vi "RIB Req - UDP Enable UPS.vi"(0 "Limits File Path":path, 5 "Results File Path":path, 11 "error in":errorcluster) -> (4 "Results Data Array":string[][](array[string]), 15 "error out":errorcluster)   [LabVIEW 2024]
doc: "Template test"
uses:
  <vilib>/addons/_JKI Toolkits/State Machine/_JKI_lib_State_Machine.llb/Select State(s)_err__jki_lib_state_machine.vi
  <vilib>/addons/_JKI Toolkits/State Machine/_JKI_lib_State_Machine.llb/Select State(s)_bool__jki_lib_state_machine.vi
  <vilib>/addons/_JKI Toolkits/State Machine/_JKI_lib_State_Machine.llb/Periodic Trigger__ogtk__JKI-SM__jki_lib_state_machine.vi
  <userlib>/_OpenG.lib/file/file.llb/Strip Path Extension - String__ogtk.vi
  <vilib>/Utility/file.llb/Read Delimited Spreadsheet (string).vi
  <userlib>/_OpenG.lib/file/file.llb/openg_file.lvlib
  <userlib>/_OpenG.lib/appcontrol/appcontrol.llb/openg_application_control.lvlib
  <userlib>/_OpenG.lib/time/time.llb/openg_time.lvlib
  <vilib>/Utility/file.llb/Write Delimited Spreadsheet (string).vi
panel:
  in  "Connect":string
  in  "Connect Fail":string
  in  "Read Normal Operation":string
  in  "Read Wait for Start":string
  in  "Read TMS":string
  in  "Read ROV B":string
  in  "Read ROV A":string
  in  "5A Test":bool
  in  "task out":refnum<k21>
  out "Timeout (Read UDP)":dbl(slide) scale=0.0..20.0
  out "Results Data 2":string[](array[string])
  in  "UDP Read":string
  in  "connection ID":refnum<k16>
  in  "Exit":bool
  # "Enable UPS Test"
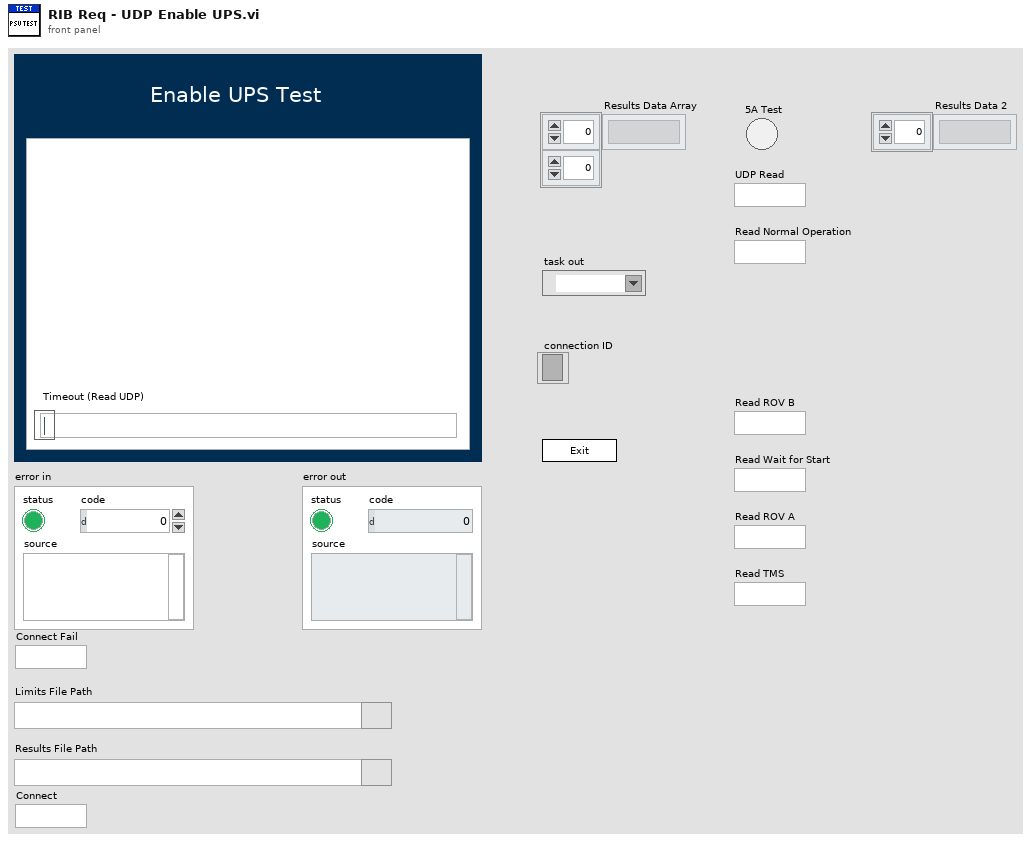
[diagram p1: front panel]
types:
  T1 = enum32{"Invalid", "Standard", "Closed", "Hidden", "Minimized", "Maximized"}
  T2 = enum32{"invalid app kind", "Development System", "Run Time System", "Student Edition", "Embedded LabVIEW", "Evaluation", "Custom"}
  T3 = typedef "FGV - Enum" = enum16{"Cleanup", "Get Data", "Open UDP", "Initialise DAQ", "Initialise I2C"}
  T4 = enum16{"Start Timer", "Get Time", "Pause", "Unpause"}
  T5 = cluster{"Core":cluster{"Current VI Reference":refnum<vi>, "Close Panel on Exit?":bool}, "Limits File Path":path, "Test Limits":string[][], "Results Data Array":string[][], "Results File Path":path, "UDP Read":string, "connection ID":refnum<k16>, "task out":refnum<k21>, "5A Test":bool, "Connect Fail":string, "Connect":string, "Read ROV A":string, "Read ROV B":string, "Read TMS":string, "Read Wait for Start":string, "Read Normal Operation":string}
  T6 = cluster{"Current VI Reference":refnum<vi>, "Close Panel on Exit?":bool}
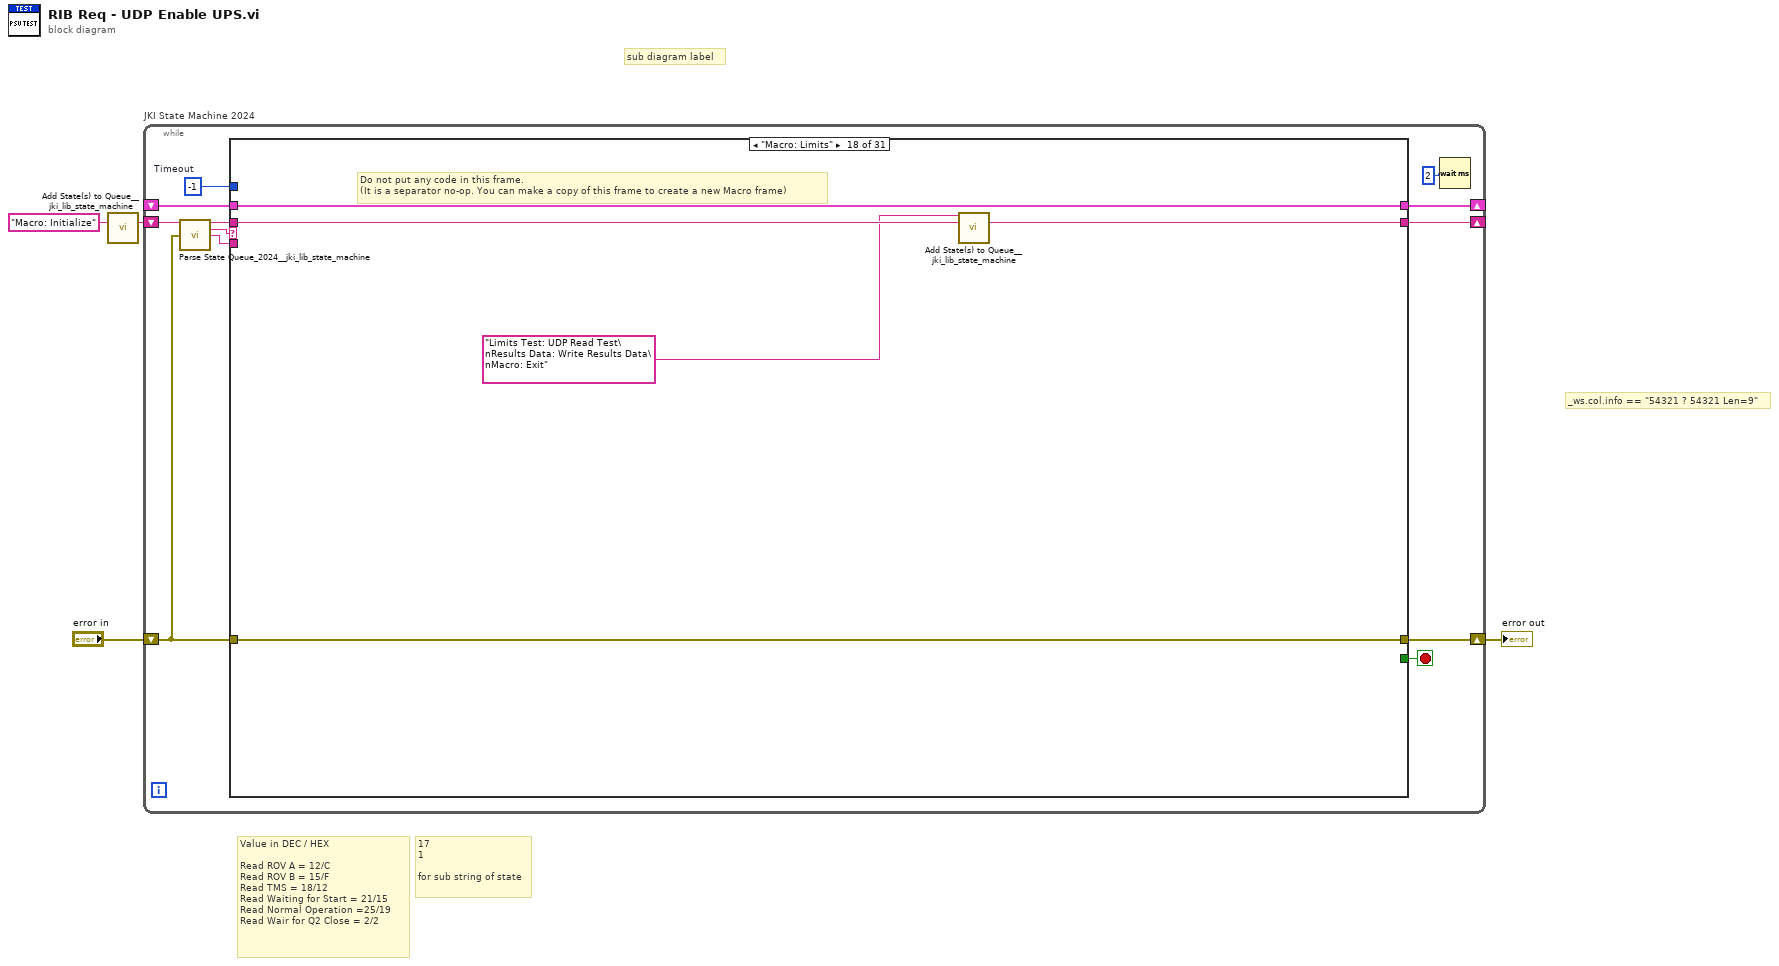
[diagram p0: block diagram]
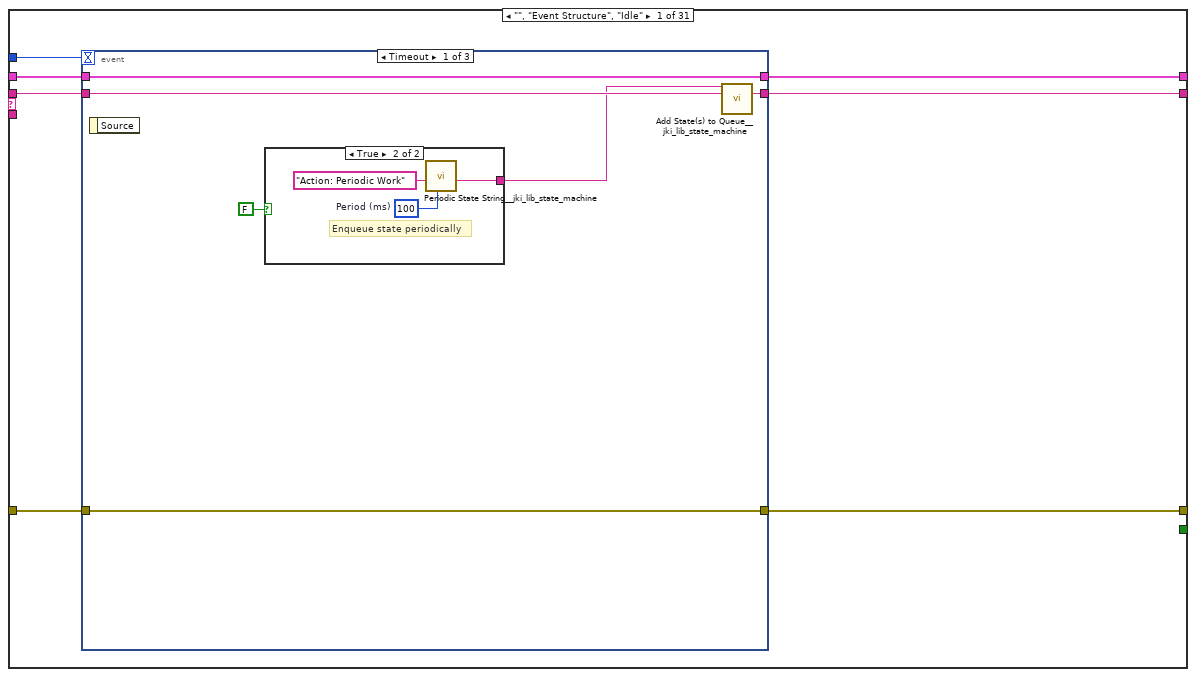
[diagram p2: hidden frame]
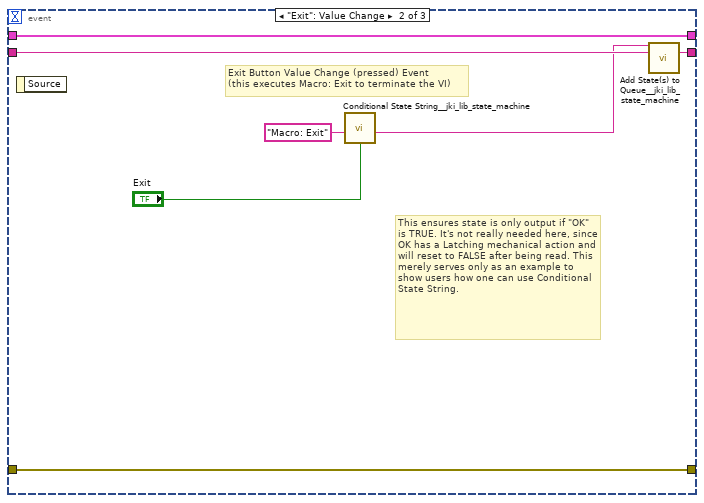
[diagram p4: hidden frame]
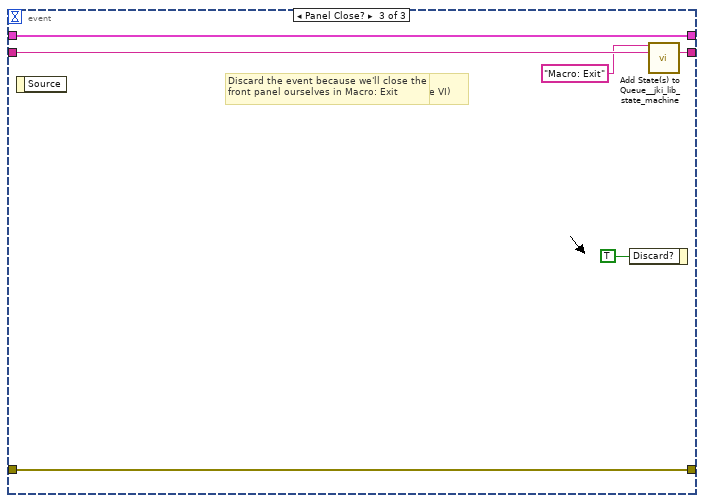
[diagram p5: hidden frame]
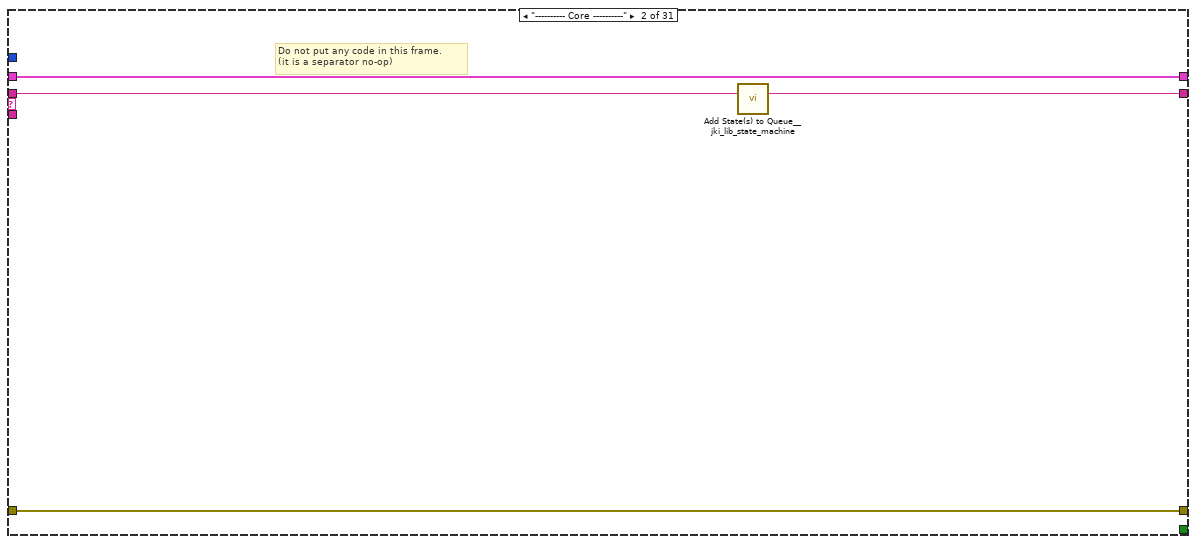
[diagram p6: hidden frame]
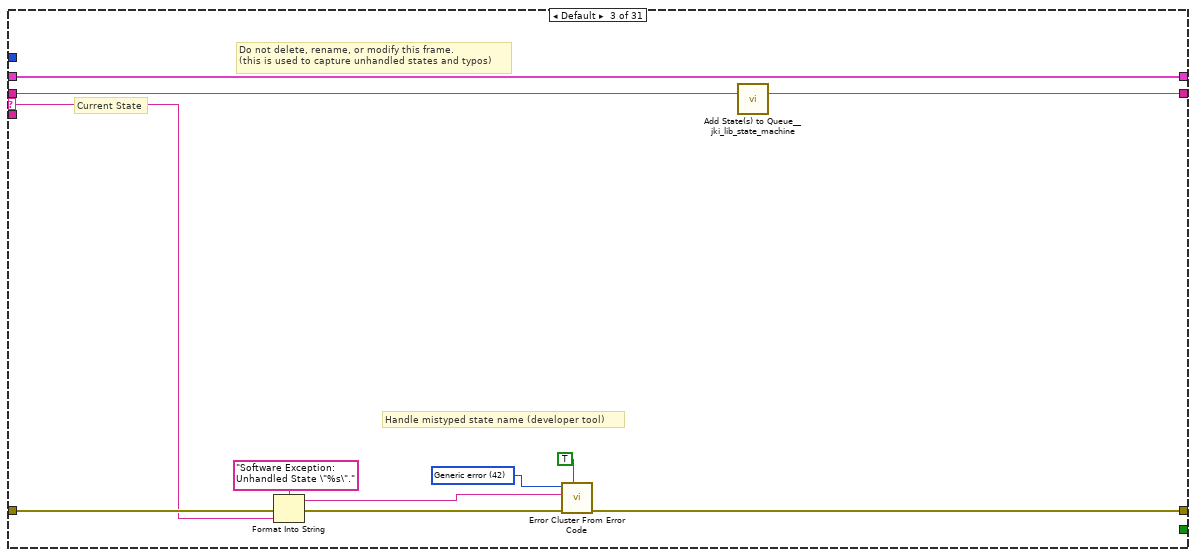
[diagram p7: hidden frame]
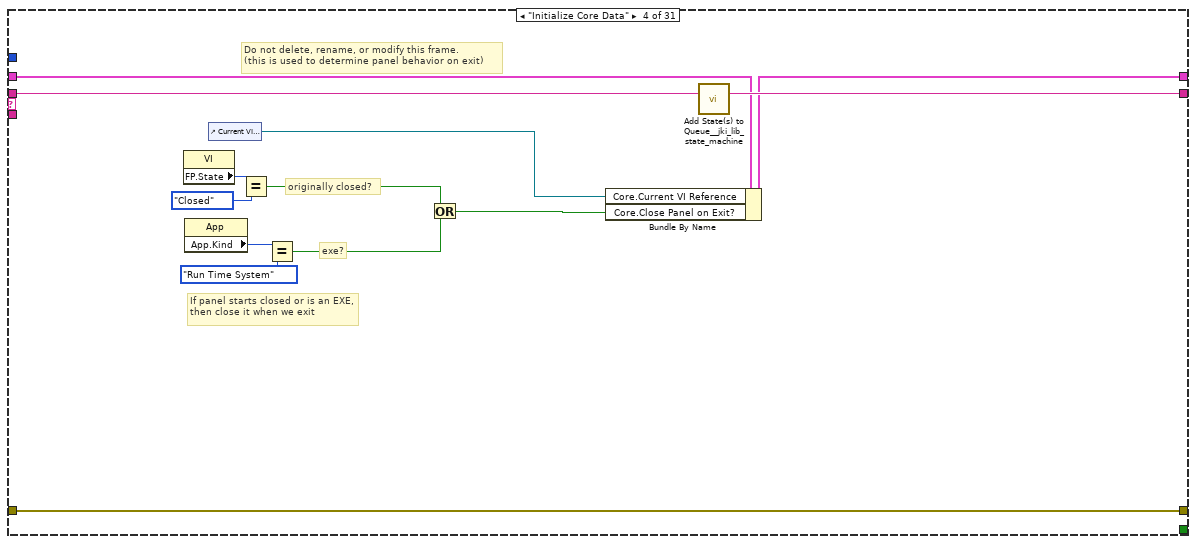
[diagram p8: hidden frame]
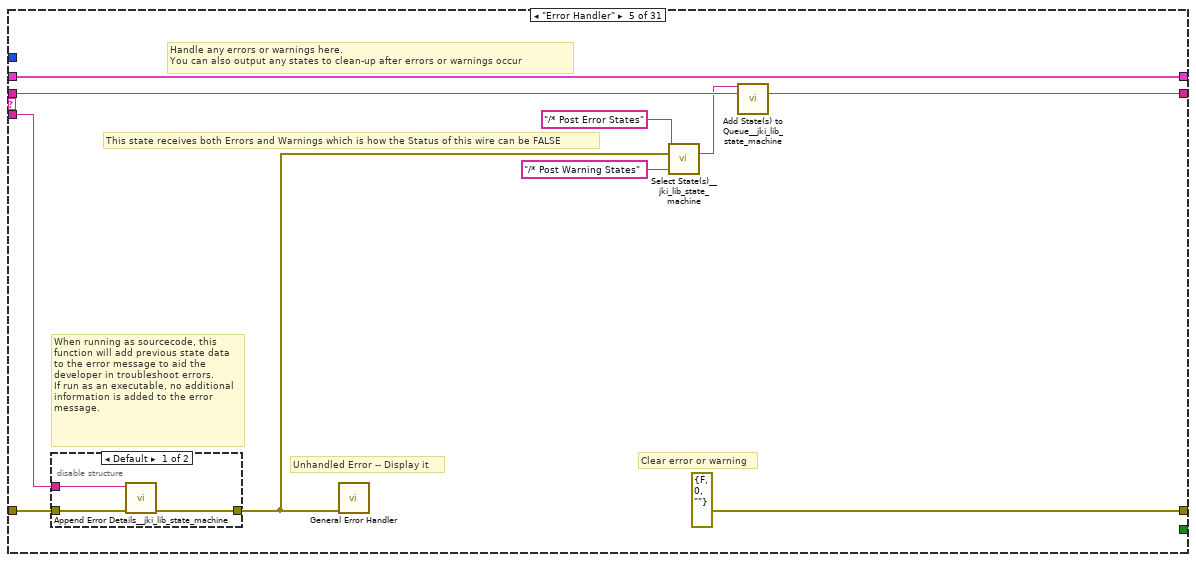
[diagram p9: hidden frame]
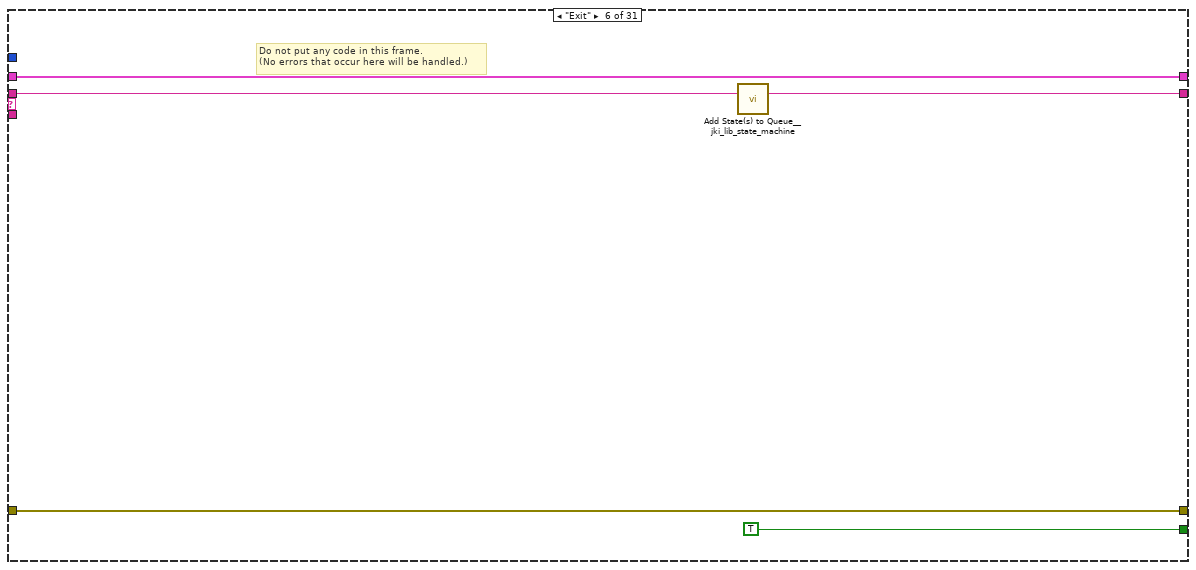
[diagram p11: hidden frame]
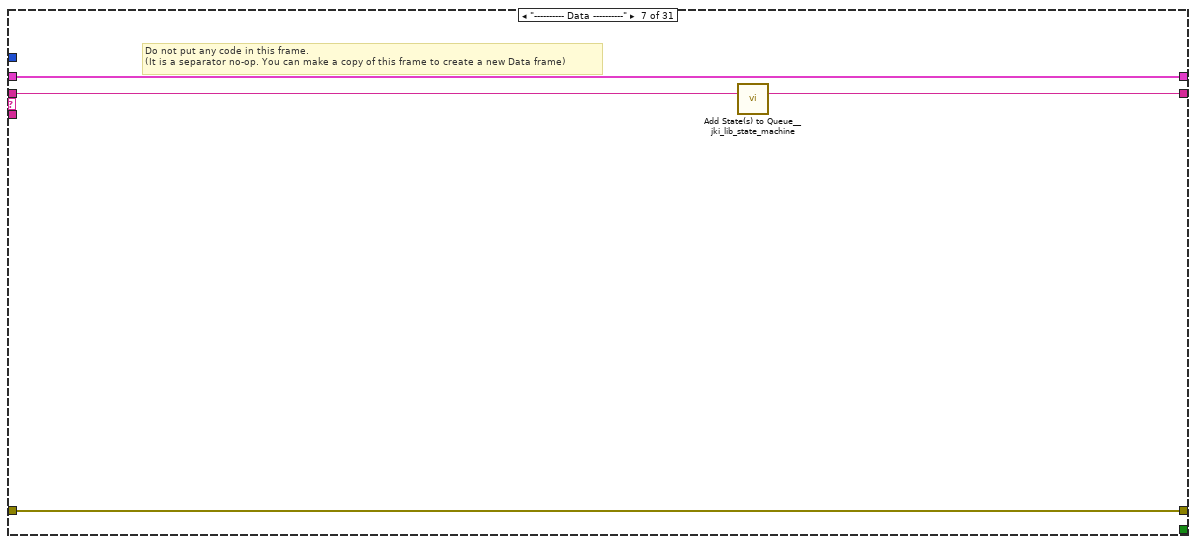
[diagram p12: hidden frame]
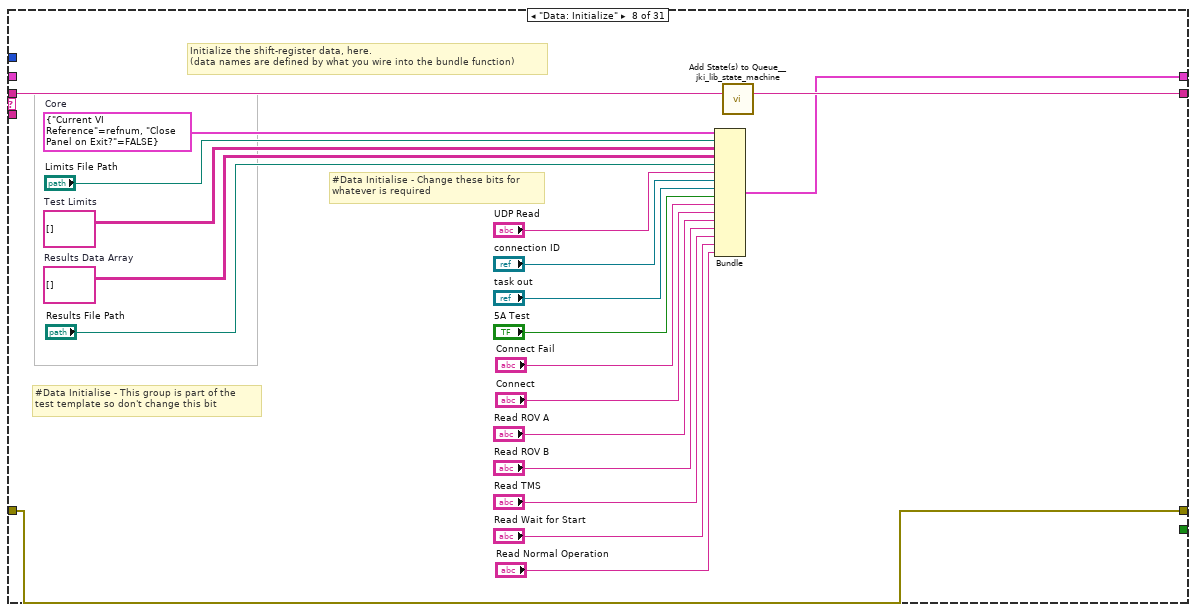
[diagram p13: hidden frame]
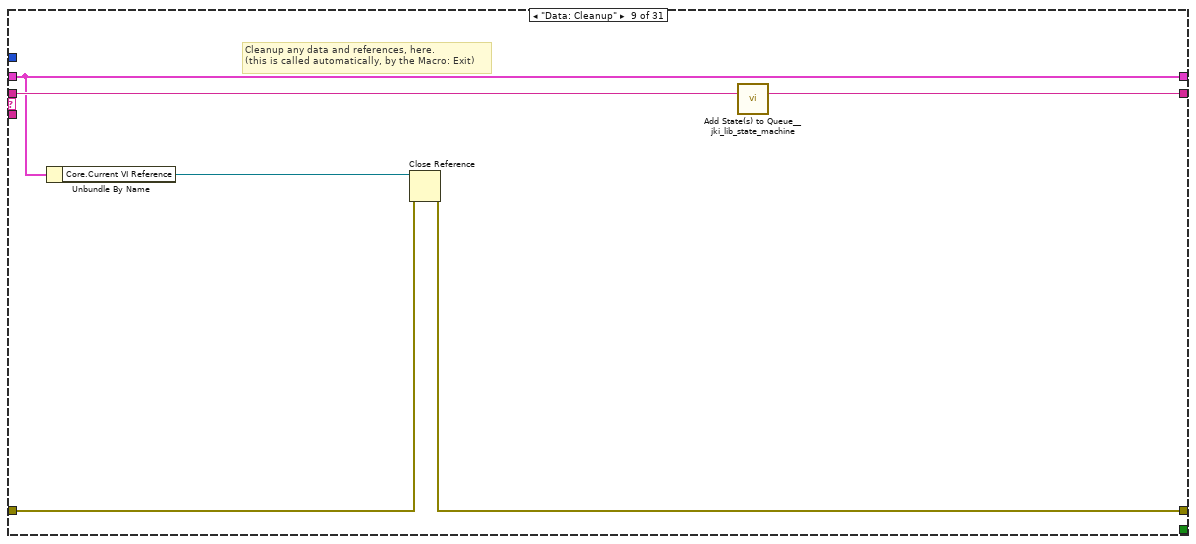
[diagram p14: hidden frame]
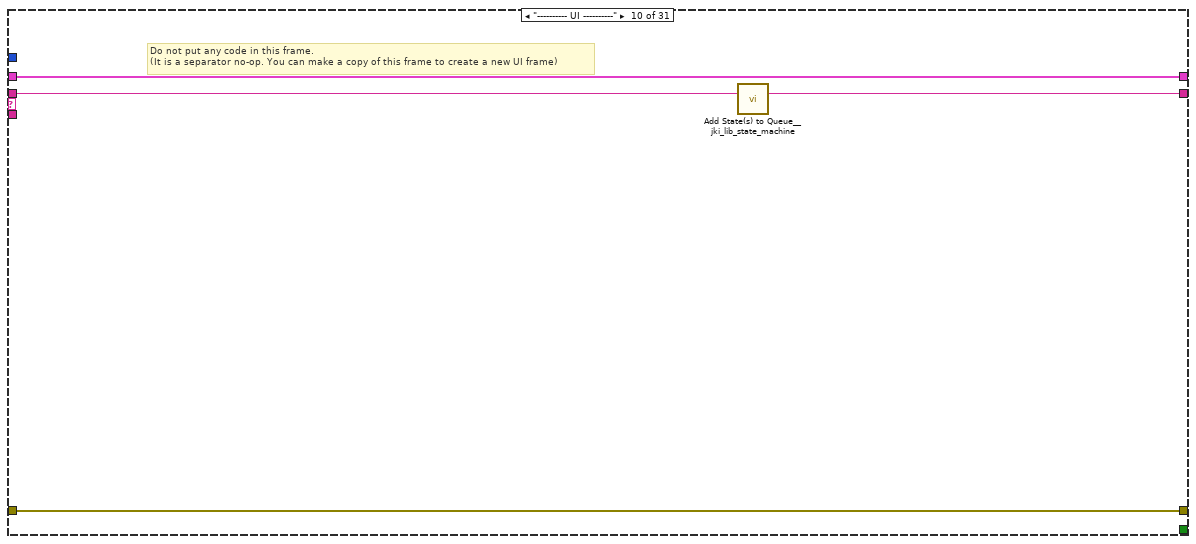
[diagram p15: hidden frame]
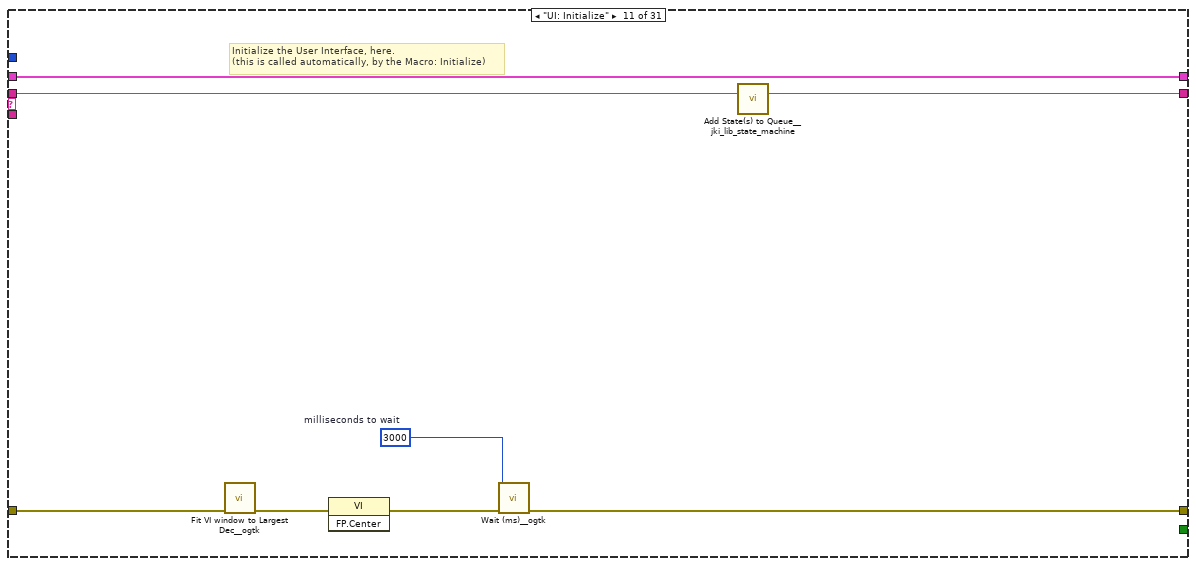
[diagram p16: hidden frame]
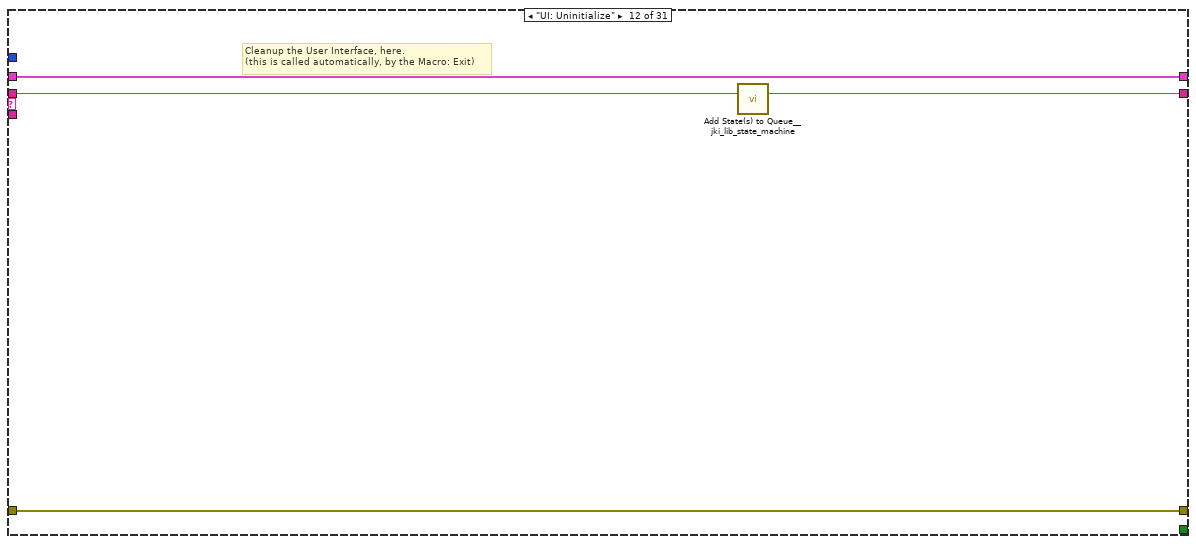
[diagram p17: hidden frame]
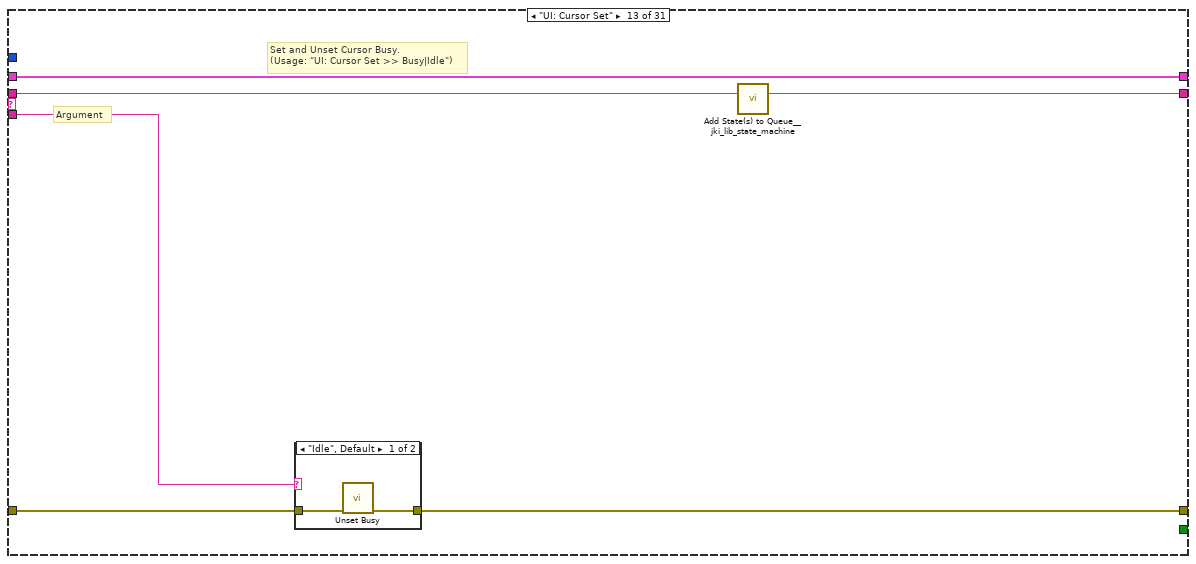
[diagram p18: hidden frame]
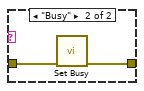
[diagram p19: hidden frame]
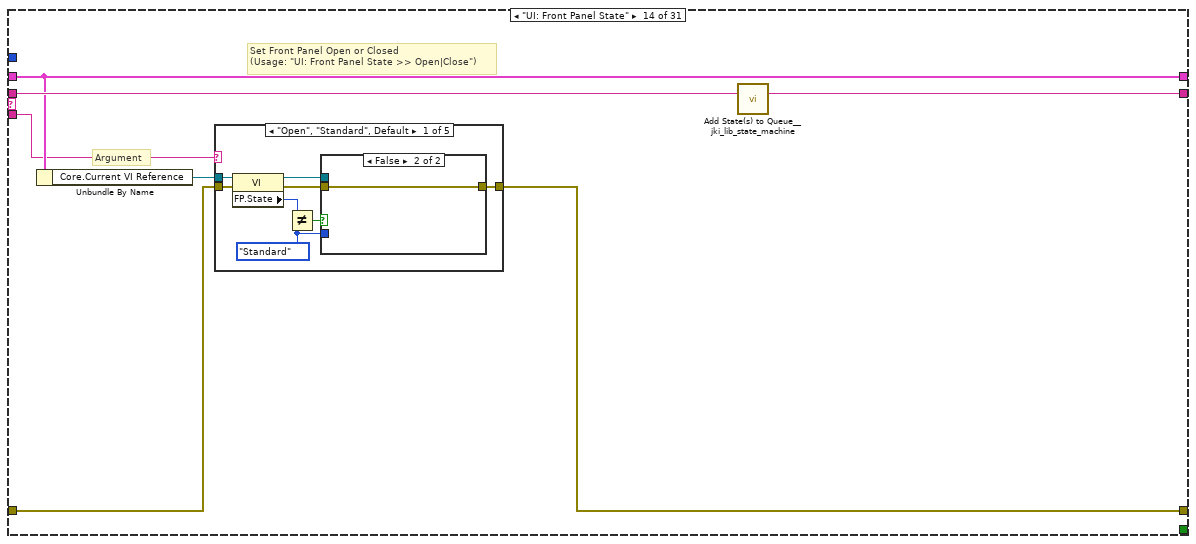
[diagram p20: hidden frame]
diagram:
  # "17\n1\n\nfor sub string of state"
  # "Value in DEC / HEX\n\nRead ROV A = 12/C\nRead ROV B = 15/F\nRead TMS = 18/12\nRead Waiting for Start = 21/15\nRead Normal Operation =25/19 \nRead Wair for Q2 Close = 2/2"
  # "_ws.col.info == \"54321 ? 54321 Len=9\""
  # "sub diagram label"
  n1 = call <vilib>:"Add State(s) to Queue__jki_lib_state_machine.vi"("State(s) in (\"\")"="Macro: Initialize") -> ("States Out"=w4:string)  [unwired: 14 in]
  n2 = while "JKI State Machine 2024" {
    shift-right: [w9] -> _
    shift-left: _ -> [w8]
    shift-right: [w12] -> w1
    shift-left: "error in" -> [w6]
    shift-right: [w11] -> _
    shift-left: w4 -> [w13]
    stop <- w10 stop-if-true
    w7 = -1  # Timeout
    n3 = call <vilib>:"Parse State Queue_2024__jki_lib_state_machine.vi"("State Queue"=w13, "Error In (no error)"=w6) -> ("Remaining States"=w15:string, "Current State"=w16:string, "Arguments"=w14:string)  [unwired: 11 in]
    n4 = case shown="\"Macro: Limits\"" w16 {
      selector: w16 -> [_ _ w50 _ _ _ _ _ _ _ _ _ _ _ _ _ _ _ _ _ _ _ _ _ _ _ _ _ _ _ _]
      tunnel: w15 -> [w23 w49 w54 w73 w83 w92 w96 w116 w122 w126 w134 w138 w144 w155 w224 w229 w234 w239 w248 w252 w265 w282 w286 w295 w299 w307 w315 w326 w346 w370 w382]
      tunnel: w14 -> [_ _ _ _ w78 _ _ _ _ _ _ _ w139 w149 _ _ _ _ _ _ _ _ _ _ _ _ _ _ _ _ _]
      tunnel: w8 -> [w21 w46 w52 w66 w80 w90 w93 _ w117 w123 w132 w136 w142 w151 w221 w226 w231 w236 w246 w249 w255 w274 w283 w291 w296 w305 w313 w324 w329 w364 w380]
      tunnel: [w20 w47 w56 w70 errorcluster {"status"=FALSE, "code"=0, "source"=""} ("error out") w89 w94 w113 w118 w124 w130 w135 w140 w152 w222 w227 w232 w237 w243 w250 w261 w279 w284 w293 w297 w302 w310 w317 w327 w350 w377] -> w12
      tunnel: w6 -> [w17 w47 w55 w70 w79 w89 w94 w113 w119 w124 w131 w135 w141 w153 w222 w227 w232 w237 w243 w250 w260 w278 w284 w292 w297 w300 w309 w322 w331 w366 w378]
      tunnel: [w22 w48 w53 w72 w82 w91 w95 w115 w121 w125 w133 w137 w143 w154 w223 w228 w233 w238 w247 w251 w264 w281 w285 w294 w298 w306 w314 w325 w345 w369 w381] -> w11
      tunnel: [_ _ _ _ _ TRUE _ _ _ _ _ _ _ _ _ _ _ _ _ _ _ _ _ _ _ _ _ _ _ _ _] -> w10
      tunnel: [w19 w46 w52 w71 w80 w90 w93 w114 w117 w123 w132 w136 w142 w151 w221 w226 w231 w236 w246 w249 w254 w273 w283 w291 w296 w304 w312 w324 w333 w363 w380] -> w9
      tunnel: w7 -> [w18 _ _ _ _ _ _ _ _ _ _ _ _ _ _ _ _ _ _ _ _ _ _ _ _ _ _ _ _ _ _]
      frame "", "Event Structure", "Idle" {
        n5 = event shown="[0] Timeout" {
          selector: _ -> [_ _ _]
          dyn-events: _ -> [_ _ _]
          timeout: w18 -> [_ _ _]
          tunnel: w23 -> [w29 w39 w45]
          tunnel: [w28 w38 w44] -> w22
          tunnel: w21 -> [w26 w36 w42]
          tunnel: [w27 w37 w43] -> w20
          tunnel: w17 -> [w27 w37 w43]
          tunnel: [w26 w36 w42] -> w19
          event Timeout {
            n6 = event-data() -> ()  [unwired: 1 in, 1 out]
            n7 = case shown="True" FALSE {
              tunnel: [_ w32] -> w25
              frame False {
              }
              frame True {
                w30 = u32 100  # Period (ms)
                # "Enqueue state periodically"
                n8 = call <vilib>:"Periodic State String__jki_lib_state_machine.vi"("Period (ms)"=w30, "State"="Action: Periodic Work") -> ("State Out"=w32:string)  [unwired: 9 in]
              }
            }
            n9 = call <vilib>:"Add State(s) to Queue__jki_lib_state_machine.vi"("State(s) in Front (\"\")"=w25, "State(s) in (\"\")"=w29) -> ("States Out"=w28:string)  [unwired: 13 in]
          }
          event "Exit": Value Change {
            # "This ensures state is only output if \"OK\" is TRUE. It's not really needed here, since OK has a Latching mechanical action and will reset to FALSE after being read. This merely serves only as an example to show users how one can use Conditional State String."
            # "Exit Button Value Change (pressed) Event\n(this executes Macro: Exit to terminate the VI)"
            n10 = event-data() -> ()  [unwired: 1 in, 1 out]
            n11 = call <vilib>:"Conditional State String__jki_lib_state_machine.vi"("Do State(s)?"="Exit", "State"="Macro: Exit") -> ("State Out"=w33:string)  [unwired: 7 in]
            n12 = call <vilib>:"Add State(s) to Queue__jki_lib_state_machine.vi"("State(s) in Front (\"\")"=w33, "State(s) in (\"\")"=w39) -> ("States Out"=w38:string)  [unwired: 13 in]
          }
          event Panel Close? {
            # "Discard the event because we'll close the front panel ourselves in Macro: Exit"
            # "Close Panel button (pressed) Event\n(this executes Macro: Exit to terminate the VI)"
            n13 = event-data() -> ()  [unwired: 1 in, 1 out]
            n14 = event-data("Discard?"=TRUE) -> ()  [unwired: 1 in, 1 out]
            n15 = call <vilib>:"Add State(s) to Queue__jki_lib_state_machine.vi"("State(s) in Front (\"\")"="Macro: Exit", "State(s) in (\"\")"=w45) -> ("States Out"=w44:string)  [unwired: 13 in]
          }
        }
      }
      frame "---------- Core ----------" {
        # "Do not put any code in this frame.\n(it is a separator no-op)"
        n16 = call <vilib>:"Add State(s) to Queue__jki_lib_state_machine.vi"("State(s) in (\"\")"=w49) -> ("States Out"=w48:string)  [unwired: 14 in]
      }
      frame Default {
        w59 = 42 items=["No error", "Argument error", "Memory is full", "Out of zone", "End of file", "File already open", "Generic file I/O error", "File not found", "File permission error", "Disk is full", "Duplicate path", "Too many files open", "System feature not enabled", "Resource file not found", "Cannot add resource", "Resource not found", "Image not found", "Image memory error", "Pen does not exist", "Config type invalid", "Config token not found", "Config parse error", "Config memory error", "Bad external code format", "Bad external code offset", "External code not present", "Null window", "Destroy window error", "Null menu", "Print aborted", "Bad print record", "Print driver error", "Windows error during printing", "Memory error during printing", "Print dialog error", "Generic print error", "Invalid device refnum", "Device not found", "Device parameter error", "Device unit error", "Cannot open device", "Device call aborted", "Generic error", "Cancelled by user", "Object ID too low", "Object ID too high", "Object not in heap", "Unknown heap", "Unknown object (invalid DefProc)", "Unknown object (DefProc not in table)", "Message out of range", "Invalid (null) method", "Unknown message", "Manager call not supported", "Bad address", "Network operation in progress", "Network operation timed out", "Connection is busy", "Network attribute not supported", "Network error", "Address in use", "System out of memory", "Connection aborted", "Connection refused", "Not connected", "Already connected", "Connection closed", "Initialization error (interapplication manager)", "Bad occurrence", "Wait on unbound occurrence handler", "Occurrence queue overflow", "Datalog type conflict", "Unused", "Unrecognized type (interapplication manager)", "Memory corrupt", "Failed to make temporary DLL", "Old CIN version", "Drag socket not found", "Failed to load drop-object", "Failed to register OLE object", "Failed to release OLE object", "Format specifier type mismatch", "Unknown format specifier", "Too few format specifiers", "Too many format specifiers", "Scan failed", "Newer CIN version", "Error converting to variant", "Runtime menu error", "Password tampered", "Variant attribute not found", "Incompatible variant data type", "Event data is not available", "Event Store is not present", "Occurrence is not found", "Event Queue is not created", "Event info is not available", "Refnum passed is NULL", "Error retrieving Class GUID", "Error retrieving CoClass GUID", "Error retrieving TypeLib GUID.", "Bad built application magic bytes.", "Specific driver is different from the specific driver associated with the Logical Name.", "There is no session opened to the class driver.", "Max Error", "MAX - Error with config objects", "MAX - Error loading configuration", "MAX - Group not supported"]
        # "Current State"
        # "Do not delete, rename, or modify this frame.\n(this is used to capture unhandled states and typos)"
        # "Handle mistyped state name (developer tool)"
        n17 = Format Into String(format string="Software Exception: Unhandled State \"%s\"." ("message"), error in=w55, w50) -> (resulting string=w58:string, error out=w57:errorcluster)  [unwired: 1 in]
        n18 = call <vilib>:"Error Cluster From Error Code.vi"("show call chain? (False)"=TRUE, "error in (no error)"=w57, "error message (\"\")"=w58, "error code (0)"=w59) -> ("error out"=w56:errorcluster)  [unwired: 5 in]
        n19 = call <vilib>:"Add State(s) to Queue__jki_lib_state_machine.vi"("State(s) in (\"\")"=w54) -> ("States Out"=w53:string)  [unwired: 14 in]
      }
      frame "Initialize Core Data" {
        # "Do not delete, rename, or modify this frame.\n(this is used to determine panel behavior on exit)"
        # "originally closed?"
        # "exe?"
        # "If panel starts closed or is an EXE, then close it when we exit"
        n20 = property class="VI"() -> ("FP.State"=w63:T1)  [unwired: 2 in, 2 out]
        n21 = property class="App"() -> ("App.Kind"=w69:T2)  [unwired: 2 in, 2 out]
        n22 = control-ref of="Current VI Reference"() -> (w64:refnum<vi>)
        n23 = Equal?(x=w63, y=T1."Closed" ("Front Panel Window:State")) -> (x = y?=w61:bool)
        n24 = Equal?(x=w69, y=T2."Run Time System" ("Application:Kind")) -> (x = y?=w67:bool)
        n25 = Or(x=w61, y=w67) -> (x .or. y?=w65:bool)
        n26 = Bundle By Name(cluster=w66, "Core.Current VI Reference"=w64, "Core.Close Panel on Exit?"=w65) -> (w71:T5)
        n27 = call <vilib>:"Add State(s) to Queue__jki_lib_state_machine.vi"("State(s) in (\"\")"=w73) -> ("States Out"=w72:string)  [unwired: 14 in]
      }
      frame "Error Handler" {
        # "When running as sourcecode, this function will add previous state data to the error message to aid the developer in troubleshoot errors.\nIf run as an executable, no additional information is added to the error message."
        # "This state receives both Errors and Warnings which is how the Status of this wire can be FALSE"
        # "Unhandled Error -- Display it"
        # "Handle any errors or warnings here.\nYou can also output any states to clean-up after errors or warnings occur"
        # "Clear error or warning"
        n28 = disable-structure shown="Default" {
          disable-tunnel: w79 -> [w86 w87]
          disable-tunnel: w78 -> [w85 _]
          disable-tunnel: [w84 w87] -> w77
          frame condition #0 (active) {
            n29 = call <vilib>:"Append Error Details__jki_lib_state_machine.vi"("error in (no error)"=w86, "Previous State and Argument(s)"=w85) -> ("error out"=w84:errorcluster)  [unwired: 9 in]
          }
          frame condition #1 {
          }
        }
        n30 = call <vilib>:"General Error Handler.vi"("error in (no error)"=w77) -> ()  [unwired: 10 in, 5 out]
        n31 = call-poly <vilib>:"Select State(s)__jki_lib_state_machine.vi"("State(s) if True (\"\")"="/* Post Error States", "Select"=w77, "State(s) if False (\"\")"="/* Post Warning States") -> ("States Out"=w75:string)  [unwired: 12 in]
        n32 = call <vilib>:"Add State(s) to Queue__jki_lib_state_machine.vi"("State(s) in Front (\"\")"=w75, "State(s) in (\"\")"=w83) -> ("States Out"=w82:string)  [unwired: 13 in]
      }
      frame "Exit" {
        # "Do not put any code in this frame.\n(No errors that occur here will be handled.)"
        n33 = call <vilib>:"Add State(s) to Queue__jki_lib_state_machine.vi"("State(s) in (\"\")"=w92) -> ("States Out"=w91:string)  [unwired: 14 in]
      }
      frame "---------- Data ----------" {
        # "Do not put any code in this frame.\n(It is a separator no-op. You can make a copy of this frame to create a new Data frame)"
        n34 = call <vilib>:"Add State(s) to Queue__jki_lib_state_machine.vi"("State(s) in (\"\")"=w96) -> ("States Out"=w95:string)  [unwired: 14 in]
      }
      frame "Data: Initialize" {
        w109 = string[][] []  # Results Data Array
        w110 = string[][] []  # Test Limits
        w112 = T6 {"Current VI Reference"=refnum, "Close Panel on Exit?"=FALSE}  # Core
        # "#Data Initialise - Change these bits for\nwhatever is required"
        # "#Data Initialise - This group is part of the\ntest template so don't change this bit"
        # "Initialize the shift-register data, here.\n(data names are defined by what you wire into the bundle function)"
        n35 = Bundle("Core"=w112, "Limits File Path"="Limits File Path", "Test Limits"=w110, "Results Data Array"=w109, "Results File Path"="Results File Path", "UDP Read"="UDP Read", "connection ID"="connection ID", "task out"="task out", "5A Test"="5A Test", "Connect Fail"="Connect Fail", "Connect"="Connect", "Read ROV A"="Read ROV A", "Read ROV B"="Read ROV B", "Read TMS"="Read TMS", "Read Wait for Start"="Read Wait for Start", "Read Normal Operation"="Read Normal Operation") -> (w114:T5)  [unwired: 1 in]
        n36 = call <vilib>:"Add State(s) to Queue__jki_lib_state_machine.vi"("State(s) in (\"\")"=w116) -> ("States Out"=w115:string)  [unwired: 14 in]
      }
      frame "Data: Cleanup" {
        # "Cleanup any data and references, here.\n(this is called automatically, by the Macro: Exit)"
        n37 = Unbundle By Name(w117) -> ("Core.Current VI Reference"=w120:refnum<vi>)
        n38 = Close Reference(reference=w120, error in (no error)=w119) -> (error out=w118:errorcluster)
        n39 = call <vilib>:"Add State(s) to Queue__jki_lib_state_machine.vi"("State(s) in (\"\")"=w122) -> ("States Out"=w121:string)  [unwired: 14 in]
      }
      frame "---------- UI ----------" {
        # "Do not put any code in this frame.\n(It is a separator no-op. You can make a copy of this frame to create a new UI frame)"
        n40 = call <vilib>:"Add State(s) to Queue__jki_lib_state_machine.vi"("State(s) in (\"\")"=w126) -> ("States Out"=w125:string)  [unwired: 14 in]
      }
      frame "UI: Initialize" {
        w129 = u32 3000  # milliseconds to wait
        # "Initialize the User Interface, here.\n(this is called automatically, by the Macro: Initialize)"
        n41 = call <userlib>:"Fit VI window to Largest Dec__ogtk.vi"("error in (no error)"=w131) -> ("error out"=w127:errorcluster)  [unwired: 5 in, 1 out]
        n42 = invoke class="VI" method="FP.Center"(error in=w127) -> (error out=w128:errorcluster)  [unwired: 2 in, 2 out]
        n43 = call <userlib>:"Wait (ms)__ogtk.vi"("error in (no error)"=w128, "milliseconds to wait"=w129) -> ("error out"=w130:errorcluster)  [unwired: 8 in, 1 out]
        n44 = call <vilib>:"Add State(s) to Queue__jki_lib_state_machine.vi"("State(s) in (\"\")"=w134) -> ("States Out"=w133:string)  [unwired: 14 in]
      }
      frame "UI: Uninitialize" {
        # "Cleanup the User Interface, here.\n(this is called automatically, by the Macro: Exit)"
        n45 = call <vilib>:"Add State(s) to Queue__jki_lib_state_machine.vi"("State(s) in (\"\")"=w138) -> ("States Out"=w137:string)  [unwired: 14 in]
      }
      frame "UI: Cursor Set" {
        # "Argument"
        # "Set and Unset Cursor Busy.\n(Usage: \"UI: Cursor Set >> Busy|Idle\")"
        n46 = case shown="\"Idle\", Default" w139 {
          tunnel: w141 -> [w146 w148]
          tunnel: [w145 w147] -> w140
          frame "Idle", Default {
            n47 = call <vilib>:"Unset Busy.vi"("error in (no error)"=w146) -> ("error out"=w145:errorcluster)  [unwired: 10 in]
          }
          frame "Busy" {
            n48 = call <vilib>:"Set Busy.vi"("error in (no error)"=w148) -> ("error out"=w147:errorcluster)  [unwired: 9 in, 1 out]
          }
        }
        n49 = call <vilib>:"Add State(s) to Queue__jki_lib_state_machine.vi"("State(s) in (\"\")"=w144) -> ("States Out"=w143:string)  [unwired: 14 in]
      }
      frame "UI: Front Panel State" {
        # "Argument"
        # "Set Front Panel Open or Closed\n(Usage: \"UI: Front Panel State >> Open|Close\")"
        n50 = Unbundle By Name(w151) -> ("Core.Current VI Reference"=w150:refnum<vi>)
        n51 = case shown="\"Open\", \"Standard\", Default" w149 {
          tunnel: w153 -> [w161 w176 w187 w200 w213]
          tunnel: [w163 w177 w189 w202 w215] -> w152
          tunnel: w150 -> [w162 w174 w188 w201 w214]
          frame "Open", "Standard", Default {
            w156 = T1."Standard" ("State")
            n52 = property class="VI"(reference=w162, error in=w161) -> (reference out=w159:refnum<vi>, error out=w160:errorcluster, "FP.State"=w158:T1)
            n53 = Not Equal?(x=w158, y=w156) -> (x != y?=w157:bool)
            n54 = case shown="False" w157 {
              tunnel: [w167 w169] -> w163
              tunnel: w160 -> [w166 w169]
              tunnel: w159 -> [w165 _]
              tunnel: w156 -> [w164 _]
              frame True {
                n55 = invoke class="VI" method="FP.Open"(reference=w165, error in=w166, "Activate"=TRUE, "State"=w164) -> (error out=w167:errorcluster)  [unwired: 1 in, 4 out]
              }
              frame False {
              }
            }
          }
          frame "Close", "Closed" {
            n56 = property class="VI"(reference=w174, error in=w176) -> (reference out=w173:refnum<vi>, error out=w175:errorcluster, "FP.State"=w171:T1)
            n57 = Not Equal?(x=w171, y=T1."Closed" ("Front Panel Window:State")) -> (x != y?=w170:bool)
            n58 = case shown="True" w170 {
              tunnel: [w178 w181] -> w177
              tunnel: w175 -> [w178 w180]
              tunnel: w173 -> [_ w179]
              frame False {
              }
              frame True {
                n59 = invoke class="VI" method="FP.Close"(reference=w179, error in=w180) -> (error out=w181:errorcluster)  [unwired: 1 in, 2 out]
              }
            }
          }
          frame "Hidden", "Hide" {
            w182 = T1."Hidden" ("State")
            n60 = property class="VI"(reference=w188, error in=w187) -> (reference out=w185:refnum<vi>, error out=w186:errorcluster, "FP.State"=w184:T1)
            n61 = Not Equal?(x=w184, y=w182) -> (x != y?=w183:bool)
            n62 = case shown="True" w183 {
              tunnel: [w193 w194] -> w189
              tunnel: w186 -> [w192 w194]
              tunnel: w185 -> [w191 _]
              tunnel: w182 -> [w190 _]
              frame True {
                n63 = invoke class="VI" method="FP.Open"(reference=w191, error in=w192, "State"=w190) -> (error out=w193:errorcluster)  [unwired: 2 in, 4 out]
              }
              frame False {
              }
            }
          }
          frame "Minimize", "Minimized" {
            w195 = T1."Minimized" ("State")
            n64 = property class="VI"(reference=w201, error in=w200) -> (reference out=w198:refnum<vi>, error out=w199:errorcluster, "FP.State"=w197:T1)
            n65 = Not Equal?(x=w197, y=w195) -> (x != y?=w196:bool)
            n66 = case shown="True" w196 {
              tunnel: [w206 w207] -> w202
              tunnel: w199 -> [w205 w207]
              tunnel: w198 -> [w204 _]
              tunnel: w195 -> [w203 _]
              frame True {
                n67 = invoke class="VI" method="FP.Open"(reference=w204, error in=w205, "State"=w203) -> (error out=w206:errorcluster)  [unwired: 2 in, 4 out]
              }
              frame False {
              }
            }
          }
          frame "Maximize", "Maximized" {
            w208 = T1."Maximized" ("State")
            n68 = property class="VI"(reference=w214, error in=w213) -> (reference out=w211:refnum<vi>, error out=w212:errorcluster, "FP.State"=w210:T1)
            n69 = Not Equal?(x=w210, y=w208) -> (x != y?=w209:bool)
            n70 = case shown="True" w209 {
              tunnel: [w219 w220] -> w215
              tunnel: w212 -> [w218 w220]
              tunnel: w211 -> [w217 _]
              tunnel: w208 -> [w216 _]
              frame True {
                n71 = invoke class="VI" method="FP.Open"(reference=w217, error in=w218, "State"=w216) -> (error out=w219:errorcluster)  [unwired: 2 in, 4 out]
              }
              frame False {
              }
            }
          }
        }
        n72 = call <vilib>:"Add State(s) to Queue__jki_lib_state_machine.vi"("State(s) in (\"\")"=w155) -> ("States Out"=w154:string)  [unwired: 14 in]
      }
      frame "---------- Macro ----------" {
        # "Do not put any code in this frame.\n(It is a separator no-op. You can make a copy of this frame to create a new Macro frame)"
        n73 = call <vilib>:"Add State(s) to Queue__jki_lib_state_machine.vi"("State(s) in (\"\")"=w224) -> ("States Out"=w223:string)  [unwired: 14 in]
      }
      frame "Macro: Initialize" {
        # "Initialization Macro\n(This is called once, when the VI starts)"
        n74 = call <vilib>:"Add State(s) to Queue__jki_lib_state_machine.vi"("State(s) in Front (\"\")"="Data: Initialize\nInitialize Core Data\nUI: Initialize\nUI: Front Panel State >> Open\nMacro: Test", "State(s) in (\"\")"=w229) -> ("States Out"=w228:string)  [unwired: 13 in]
      }
      frame "Macro: Test" {
        # "#Test Macro - Add the sequence \nfor measurments and limits testing here"
        n75 = call <vilib>:"Add State(s) to Queue__jki_lib_state_machine.vi"("State(s) in Front (\"\")"="Limits Test: Read Limits File\nEnable UPS: UDP Open\nEnable UPS: I2C Open\nEnable UPS: Start Timer\nEnable UPS: UPD Enable UPS\nEnable UPS: Read UDP", "State(s) in (\"\")"=w234) -> ("States Out"=w233:string)  [unwired: 13 in]
      }
      frame "Macro: Limits" {
        # "Do not put any code in this frame.\n(It is a separator no-op. You can make a copy of this frame to create a new Macro frame)"
        n76 = call <vilib>:"Add State(s) to Queue__jki_lib_state_machine.vi"("State(s) in Front (\"\")"="Limits Test: UDP Read Test\nResults Data: Write Results Data\nMacro: Exit", "State(s) in (\"\")"=w239) -> ("States Out"=w238:string)  [unwired: 13 in]
      }
      frame "Macro: Exit" {
        # "Exit Macro\n(This is called once, when the VI exits)"
        n77 = Unbundle By Name(w246) -> ("Core.Close Panel on Exit?"=w241:bool)
        n78 = call <vilib>:"Conditional State String__jki_lib_state_machine.vi"("Do State(s)?"=w241, "State"="UI: Front Panel State >> Close") -> ("State Out"=w240:string)  [unwired: 7 in]
        n79 = call <vilib>:"Add State(s) to Queue__jki_lib_state_machine.vi"("State(s) in (\"\")"=w240, "State(s) at Back (\"\")"="UI: Uninitialize\nData: Cleanup\nExit") -> ("States Out"=w244:string)  [unwired: 13 in]
        n80 = call <vilib>:"Add State(s) to Queue__jki_lib_state_machine.vi"("State(s) in Front (\"\")"=w244, "State(s) in (\"\")"=w248) -> ("States Out"=w247:string)  [unwired: 13 in]
      }
      frame "---------- Limits Test ----------" {
        # "Template Separator\n(You can make a copy of, or modify, this frame)"
        n81 = call <vilib>:"Add State(s) to Queue__jki_lib_state_machine.vi"("State(s) in (\"\")"=w252) -> ("States Out"=w251:string)  [unwired: 14 in]
      }
      frame "Limits Test: Read Limits File" {
        w258 = ","  # delimiter (\t)
        n82 = Unbundle By Name(w255) -> ("Limits File Path"=w259:path)
        n83 = Current VI's Path "Test Case Path"() -> (path=w263:path)
        n84 = call-poly <vilib>:"Read Delimited Spreadsheet.vi"("file path (dialog if empty)"=w259, "error in (no error)"=w260, "delimiter (\\t)"=w258) -> ("all rows"=w256:string[][], "error out"=w261:errorcluster)  [unwired: 7 in, 4 out]
        n85 = Strip Path(path=w263) -> (name=w262:string)  [unwired: 1 out]
        n86 = call-poly <userlib>:"Strip Path Extension__ogtk.vi"("path"=w262) -> ("root"=w257:string)  [unwired: 1 out]
        n87 = for {
          tunnel: w257 -> [w269]
          tunnel: w256 -> [w267] mode=indexing
          tunnel: [w267] -> w253 mode=indexing if=w266
          n88 = Index Array(array=w267) -> (element=w268:string)  [unwired: 1 in]
          n89 = Equal?(x=w269, y=w268) -> (x = y?=w266:bool)
        }
        n90 = Bundle By Name(cluster=w255, "Test Limits"=w253) -> (w254:T5)
        n91 = call <vilib>:"Add State(s) to Queue__jki_lib_state_machine.vi"("State(s) in (\"\")"=w265) -> ("States Out"=w264:string)  [unwired: 14 in]
      }
      frame "Limits Test: UDP Read Test" {
        w275 = "UDP Read Test"  # Sub Test Name
        # "UDP Read Test = if equal to F0 = pass else fail"
        # "#Limits Testing - Add the sub test name for\ntest included in limits file"
        n92 = Unbundle By Name(w274) -> ("Results Data Array"=w272:string[][])
        n93 = Unbundle By Name(w274) -> ("Test Limits"=w276:string[][], "UDP Read"=w280:string)
        n94 = To Variant(anything=w280) -> (Variant=w277:variant)
        n95 = call "Process Results.vi"("error in (no error)"=w278, "Measurement"=w277, "Test Limits"=w276, "Sub Test Name"=w275) -> ("error out"=w279:errorcluster, "Results Data"=w270:string[])  [unwired: 6 in]
        "Results Data 2" <- w270
        n96 = Build Array (concatenate)(w272, w270) -> (w271:string[][])
        n97 = Bundle By Name(cluster=w274, "Results Data Array"=w271) -> (w273:T5)
        n98 = call <vilib>:"Add State(s) to Queue__jki_lib_state_machine.vi"("State(s) in (\"\")"=w282) -> ("States Out"=w281:string)  [unwired: 14 in]
      }
      frame "---------- Results Data ----------" {
        # "Template Separator\n(You can make a copy of, or modify, this frame)"
        n99 = call <vilib>:"Add State(s) to Queue__jki_lib_state_machine.vi"("State(s) in (\"\")"=w286) -> ("States Out"=w285:string)  [unwired: 14 in]
      }
      frame "Results Data: Write Results Data" {
        w288 = ","  # delimiter (\t)
        w289 = TRUE  # append to file? (new file:F)
        n100 = Unbundle By Name(w291) -> ("Results File Path"=w290:path, "Results Data Array"=w287:string[][])
        "Results Data Array" <- w287
        n101 = call-poly <vilib>:"Write Delimited Spreadsheet.vi"("file path (dialog if empty)"=w290, "2D data"=w287, "append to file? (new file:F)"=w289, "error in (no error)"=w292, "delimiter (\\t)"=w288) -> ("error out"=w293:errorcluster)  [unwired: 9 in, 1 out]
        n102 = call <vilib>:"Add State(s) to Queue__jki_lib_state_machine.vi"("State(s) in (\"\")"=w295) -> ("States Out"=w294:string)  [unwired: 14 in]
      }
      frame "---------- Enable UPS ----------" {
        # "Template Separator\n(You can make a copy of, or modify, this frame)"
        n103 = call <vilib>:"Add State(s) to Queue__jki_lib_state_machine.vi"("State(s) in (\"\")"=w299) -> ("States Out"=w298:string)  [unwired: 14 in]
      }
      frame "Enable UPS: UDP Open" {
        # "Template Separator\n(You can make a copy of, or modify, this frame)"
        # "Open UDP linking to RIB Box."
        n104 = call "FGV - Initialise.vi"("Enum"=FGV_-_Enum."Get Data", "Error In"=w300) -> ("connection ID"=w301:refnum<k16>, "Error Out"=w302:errorcluster)  [unwired: 10 in, 2 out]
        n105 = Bundle By Name(cluster=w305, "connection ID"=w301) -> (w304:T5)
        n106 = call <vilib>:"Add State(s) to Queue__jki_lib_state_machine.vi"("State(s) in (\"\")"=w307) -> ("States Out"=w306:string)  [unwired: 14 in]
      }
      frame "Enable UPS: I2C Open" {
        # "Template Separator\n(You can make a copy of, or modify, this frame)"
        n107 = call "FGV - Initialise.vi"("Enum"=FGV_-_Enum."Get Data", "Error In"=w309) -> ("task out"=w308:refnum<k21>, "Error Out"=w310:errorcluster)  [unwired: 10 in, 2 out]
        n108 = Bundle By Name(cluster=w313, "task out"=w308) -> (w312:T5)
        n109 = call <vilib>:"Add State(s) to Queue__jki_lib_state_machine.vi"("State(s) in (\"\")"=w315) -> ("States Out"=w314:string)  [unwired: 14 in]
      }
      frame "Enable UPS: Start Timer" {
        # "Start 10 second timer"
        # "Template Separator\n(You can make a copy of, or modify, this frame)"
        n110 = call "Timer.vi"("error in (no error)"=w322, "Enum"=T4."Start Timer") -> ("error out"=w321:errorcluster)  [unwired: 6 in, 3 out]
        n111 = property on="Timeout (Read UDP)" class="Slide (strict)"(error in=w321, "Value"=0.0 ("Horizontal Pointer Slide"), "Scale.Maximum"=20.0 ("Target Time"), "Scale.Minimum"=0.0 ("Scale.Range:Minimum")) -> (error out=w317:errorcluster)  [unwired: 1 in, 1 out]
        n112 = call <vilib>:"Add State(s) to Queue__jki_lib_state_machine.vi"("State(s) in Front (\"\")"="Enable UPS: UPD Enable UPS" ("State(s) in Front (\"\")"), "State(s) in (\"\")"=w326) -> ("States Out"=w325:string)  [unwired: 13 in]
      }
      frame "Enable UPS: UPD Enable UPS" {
        # "Send Enable UPS command to RIB Box"
        # "ENABLE UPS"
        # "Template Separator\n(You can make a copy of, or modify, this frame)"
        n113 = Unbundle By Name(w329) -> ("connection ID"=w328:refnum<k16>)
        n114 = Build Array(u8 91 ("element"), u8 1 ("element"), u8 9 ("element"), u8 112 ("element"), u8 1 ("element"), u8 1 ("element")) -> (w343:u8[])
        n115 = String To IP(1:"192.168.201.21" ("name")) -> (0:w336:u32)
        n116 = Byte Array To String(unsigned byte array=w343) -> (string=w337:string)
        n117 = UDP Write(address=w336, port or service name=u16 54321, connection ID=w328, data in=w337, 8:w331, 9:1000 ("timeout ms (25000)")) -> (error out=w327:errorcluster, 3:w332:refnum<k16>)
        n118 = Bundle By Name(cluster=w329, "connection ID"=w332) -> (w333:T5)
        n119 = call <vilib>:"Add State(s) to Queue__jki_lib_state_machine.vi"("State(s) in (\"\")"=w346) -> ("States Out"=w345:string)  [unwired: 14 in]
      }
      frame "Enable UPS: Read UDP" {
        # "Read UDP if equal to F0 test complete if not check if timer has elapsed."
        # "#56 = didnt read before the timeout"
        # "Template Separator\n(You can make a copy of, or modify, this frame)"
        n120 = Unbundle By Name(w364) -> ("connection ID"=w365:refnum<k16>)
        n121 = UDP Read(connection ID=w365, timeout ms (25000)=10, 8:w366) -> (data out=w352:string, error out=w351:errorcluster, 3:w347:refnum<k16>)  [unwired: 1 in, 2 out]
        n122 = String Subset(string=w352, offset (0)=81 ("offset (0) 2"), length (rest)=1 ("length (rest) 2")) -> (substring=w359:string)
        n123 = String To Byte Array(string=w359) -> (unsigned byte array=w362:u8[])
        n124 = Number To Hexadecimal String(2:w362) -> (0:w361:string[])  [unwired: 1 in]
        n125 = Index Array(array=w361, index=0) -> (element=w348:string)
        n126 = call <vilib>:"Clear Errors.vi"("error in (no error)"=w351, "specific error code to clear (0: all)"=56) -> ("error out"=w350:errorcluster)  [unwired: 4 in, 1 out]
        n127 = Equal?(x=w348, y="F0") -> (x = y?=w356:bool)
        n128 = Bundle By Name(cluster=w364, "connection ID"=w347, "UDP Read"=w348) -> (w363:T5)
        n129 = call-poly <vilib>:"Select State(s)__jki_lib_state_machine.vi"("State(s) if True (\"\")"="Macro: Limits" ("State(s) if True (\"\")"), "Select"=w356, "State(s) if False (\"\")"="Enable UPS: Elapsed Timer" ("State(s) if False (\"\")")) -> ("States Out"=w354:string)  [unwired: 12 in]
        n130 = call <vilib>:"Add State(s) to Queue__jki_lib_state_machine.vi"("State(s) in Front (\"\")"=w354, "State(s) in (\"\")"=w370) -> ("States Out"=w369:string)  [unwired: 13 in]
      }
      frame "Enable UPS: Elapsed Timer" {
        # "check if timer elased - if TRUE end test if FALSE read again."
        # "Template Separator\n(You can make a copy of, or modify, this frame)"
        # "Check to see if the timer has elpased."
        n131 = call "Timer.vi"("error in (no error)"=w378, "Target Time"=20.0, "Enum"=T4."Get Time") -> ("error out"=w377:errorcluster, "Time Elapsed?"=w374:bool, "Elapsed Time"=→"Timeout (Read UDP)":dbl)  [unwired: 5 in, 1 out]
        n132 = call-poly <vilib>:"Select State(s)__jki_lib_state_machine.vi"("State(s) if True (\"\")"="Macro: Limits" ("State(s) if True (\"\")"), "Select"=w374, "State(s) if False (\"\")"="Enable UPS: Read UDP" ("State(s) if False (\"\")")) -> ("States Out"=w373:string)  [unwired: 12 in]
        n133 = call <vilib>:"Add State(s) to Queue__jki_lib_state_machine.vi"("State(s) in Front (\"\")"=w373, "State(s) in (\"\")"=w382) -> ("States Out"=w381:string)  [unwired: 13 in]
      }
    }
    n134 = Wait (ms)(milliseconds to wait=u32 2) -> ()  [unwired: 1 out]
  }
  "error out" <- w1
